vi "Decode.vi"(10 "Encoded String":string, 11 "CfgEncoding in":refnum<class "Encoding.lvclass">) -> (2 "String":string, 3 "CfgEncoding out":refnum<class "Encoding.lvclass">)   [LabVIEW 2013, in "CfgManager.lvlib" / "Encoding.lvclass"]
uses:
  Encoding.lvclass
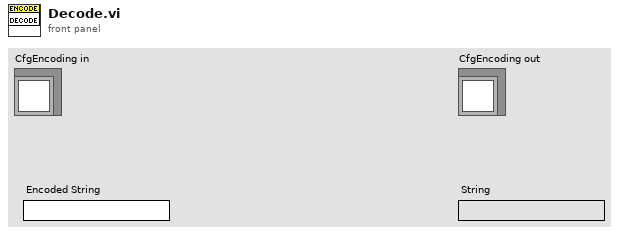
[diagram p1: front panel]
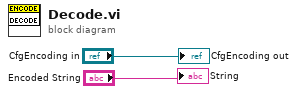
[diagram p0: block diagram]
diagram:
  "CfgEncoding out" <- "CfgEncoding in"
  "String" <- "Encoded String"
